vi "Problem 1.vi"() -> ()   [LabVIEW 2025]
panel:
  out "sum":i32
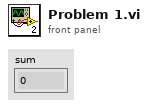
[diagram p1: front panel]
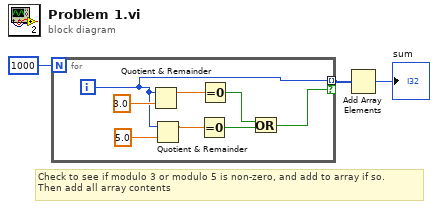
[diagram p0: block diagram]
diagram:
  # "Check to see if modulo 3 or modulo 5 is non-zero, and add to array if so. \nThen add all array contents"
  n1 = for {
    N: 1000 -> [_]
    tunnel: [w5] -> w2 mode=indexing if=w4
    i -> [w5]
    n2 = Quotient & Remainder(x=w5, y=3.0) -> (x-y*floor(x/y)=w10:dbl)  [unwired: 1 out]
    n3 = Quotient & Remainder(x=w5, y=5.0) -> (x-y*floor(x/y)=w8:dbl)  [unwired: 1 out]
    n4 = Equal To 0?(x=w8) -> (x = 0?=w6:bool)
    n5 = Equal To 0?(x=w10) -> (x = 0?=w7:bool)
    n6 = Or(x=w7, y=w6) -> (x .or. y?=w4:bool)
  }
  n7 = Add Array Elements(numeric array=w2) -> (sum=→"sum":i32)
